vi "[Comment] Input.vi"() -> (14 "Comment out":string, 15 "Canceled?":bool)   [LabVIEW 2019, in "Graph Tools.lvlib"]
uses:
  Graph Tools.lvlib
panel:
  in  "Cancel":bool
  in  "OK":bool
  in  "Write Comment":string
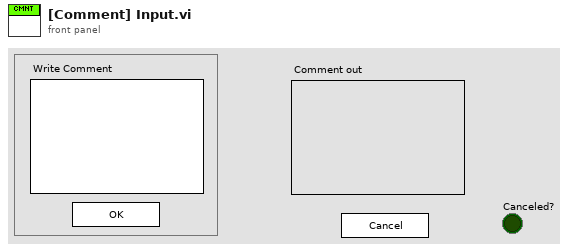
[diagram p1: front panel]
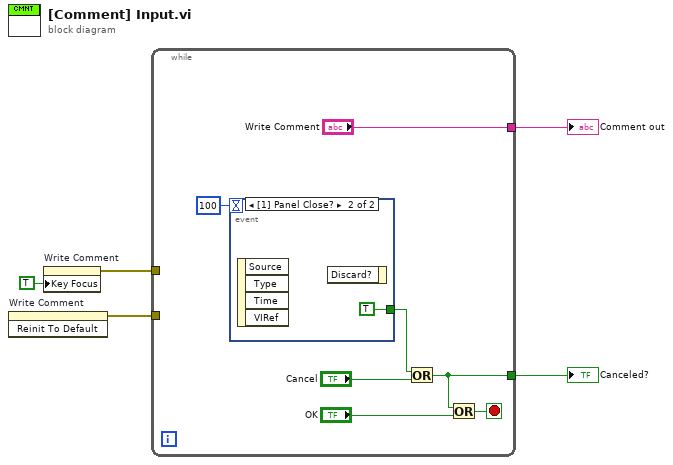
[diagram p0: block diagram]
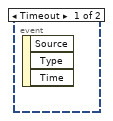
[diagram p2: hidden frame]
diagram:
  n1 = invoke on="Write Comment" class="Str" method="Reinit To Default"() -> (error out=w2:errorcluster)  [unwired: 3 in, 2 out]
  n2 = property on="Write Comment" class="Str"("Key Focus"=TRUE) -> (error out=w1:errorcluster)  [unwired: 2 in, 1 out]
  n3 = while {
    tunnel: [w7] -> w4
    tunnel: ["Write Comment"] -> w3
    tunnel: w2 -> [_]
    tunnel: w1 -> [_]
    stop <- w10 stop-if-true
    n4 = event shown="[1] Panel Close?" {
      selector: _ -> [_ _]
      dyn-events: _ -> [_ _]
      timeout: 100 -> [_ _]
      tunnel: [_ TRUE ("x")] -> w6
      event Timeout {
        n5 = event-data() -> ()  [unwired: 1 in, 3 out]
      }
      event Panel Close? {
        n6 = event-data() -> ()  [unwired: 1 in, 4 out]
        n7 = event-data() -> ()  [unwired: 2 in, 1 out]
      }
    }
    n8 = Or(x=w6, y="Cancel") -> (x .or. y?=w7:bool)
    n9 = Or(x=w7, y="OK") -> (x .or. y?=w10:bool)
  }
  "Canceled?" <- w4
  "Comment out" <- w3
